vi "FPGA Combined.vi"() -> ()   [LabVIEW 2017]
uses:
  <vilib>/ni/Engine Simulation Toolkit (EST)/Version Token.ctl
  <vilib>/ni/Engine Simulation Toolkit (EST)/APU/Settings.ctl
  <vilib>/ni/Engine Simulation Toolkit (EST)/APU/Input.ctl
  <vilib>/ni/Engine Simulation Toolkit (EST)/APU/Output.ctl
  <vilib>/ni/Engine Simulation Toolkit (EST)/Analog Replay/Settings.ctl
  <vilib>/ni/Engine Simulation Toolkit (EST)/Analog Replay/Input.ctl
  <vilib>/ni/Engine Simulation Toolkit (EST)/Analog Replay/Load Input.ctl
  <vilib>/ni/Engine Simulation Toolkit (EST)/Digital Pattern Generation/Load Input.ctl
  <vilib>/ni/Engine Simulation Toolkit (EST)/Digital Pattern Generation/Settings.ctl
  <vilib>/ni/Engine Simulation Toolkit (EST)/Digital Pattern Generation/Input.ctl
  <vilib>/ni/Engine Simulation Toolkit (EST)/APU/Shared Settings.ctl
  Documents/github/NIVeristandAdd-ons/FPGA-Custom-Device/Source/FPGA/Speciality IO/Types/PWM.Generate.Digital.Settings.ctl
  Documents/github/NIVeristandAdd-ons/FPGA-Custom-Device/Source/FPGA/Speciality IO/Types/PWM.Measure.Digital.Settings.ctl
  Documents/github/NIVeristandAdd-ons/FPGA-Custom-Device/Source/FPGA/Speciality IO/Types/PWM.Measure.Digital.Measurement.ctl
  Documents/github/NIVeristandAdd-ons/FPGA-Custom-Device/Source/FPGA/Speciality IO/Types/Sine.Generate.Settings.ctl
  Documents/github/NIVeristandAdd-ons/FPGA-Custom-Device/Source/FPGA/Speciality IO/Types/PWM.Measure.Analog.Settings.ctl
  Documents/github/NIVeristandAdd-ons/FPGA-Custom-Device/Source/FPGA/Speciality IO/Types/PWM.Measure.Analog.Measurement.ctl
  <vilib>/Platform/TimedLoop/XDataNode/timing_clust.ctl
  <vilib>/Platform/TimedLoop/XDataNode/nitl_modes.ctl
  <vilib>/Platform/TimedLoop/XDataNode/wakeup.ctl
  <vilib>/rvi/Emulation/niFpgaGetClockAttributes.vi
  <vilib>/rvi/Emulation/niFpgaSctlEmulationGetInTimedLoop.vi
  <vilib>/rvi/Emulation/niFpgaEmulationReportErrorSimple.vi
  <vilib>/rvi/DataTransferAndStorage/Container/Common/niFpgaContainerGetUniqueNameForEmu.vi
  <vilib>/rvi/DataTransferAndStorage/Container/Common/niFpgaContainerSetEmuInfo.vi
  <vilib>/rvi/eio/common/nirviEmuReportErrorAndStop.vi
  <vilib>/rvi/Emulation/niFpgaCriticalErrorInLSC.vi
  <vilib>/rvi/eio/common/nirviEmuTemplateMethod_errors.vi
  <vilib>/rvi/Emulation/niFpgaProcessEmulError.vi
  <vilib>/Platform/TimedLoop/XDataNode/XDataNode.xnode
  <vilib>/rvi/LocalResourceManager/LocalResourceManager.xnode
  <vilib>/eio/EIONode/EIONode.xnode
  <vilib>/eio/EIOMethodNode/EIOMethodNode.xnode
  <vilib>/Platform/TimedLoop/XDataNode/XDNodeRunTimeDep.lvlib
  <vilib>/ni/Engine Simulation Toolkit (EST)/APU/APU.lvlib
  <vilib>/ni/Engine Simulation Toolkit (EST)/Analog Replay/Analog Replay.lvlib
  <vilib>/ni/Engine Simulation Toolkit (EST)/Digital Pattern Generation/Digital Pattern Generation.lvlib
  Documents/github/NIVeristandAdd-ons/FPGA-Custom-Device/Source/FPGA/Speciality IO/Speciality FPGA IO.lvlib
  <vilib>/NI Veristand/FPGA/NI_VS FPGA Support.lvlib
  <vilib>/ni/Engine Simulation Toolkit (EST)/Engine Simulation Toolkit.lvlib
panel:
  in  "_Low Pulse 0":u32
  in  "_High Pulse 0":u32
  in  "_Low Pulse 1":u32
  in  "_High Pulse 1":u32
  in  "_PWM In 0 timeout":u32=40000
  out "_PWM In 0 High Time":u32
  out "_PWM In 0 Low Time":u32
  in  "_PWM In 1 timeout":u32=40000
  out "_PWM In 1 High Time":u32
  out "_PWM In 1 Low Time":u32
  in  "Generate IRQ":bool
  in  "Clock Pulse":bool
  in  "Clock Ticked":bool
  in  "Use External Timing":bool
  in  "Write to  RTSI":bool
  in  "Loop Rate (usec)":u32
  in  "Start":bool
  out "Measure.Analog.Ch0":T1={"ACTIVE TICKS"=10, "INACTIVE TICKS"=10, "ACQ TICKS"=400, "ACTIVE VOLTAGE"=4.979251861572266, "INACTIVE VOLTAGE"=-4.979404449462891}
  out "Measure.Analog.Ch1":T1={"ACTIVE TICKS"=90, "INACTIVE TICKS"=10, "ACQ TICKS"=400, "ACTIVE VOLTAGE"=-6.998723030090332, "INACTIVE VOLTAGE"=6.998509407043457}
  in  "Measure.Analog.Ch0.Settings":T2={"ACTIVE EDGE"=TRUE, "TIMEOUT"=40000000, "THRESHOLD"=0.0}
  in  "Measure.Analog.Ch1.Settings":T2={"ACTIVE EDGE"=FALSE, "TIMEOUT"=40000000, "THRESHOLD"=95.0}
  out "Analog.Generation.Ticks 2":u32=10 caption="Count(uSec)"
  in  "Analog.Generation.Ticks":u32=10 caption="Count(uSec)"
  in  "Sine":bool=TRUE
  in  "Generate.Sine.Ch0.Settings":T3
  in  "Generate.Sine.Ch1.Settings":T3
  out "Measure.Digital.Ch0":T4={"ACTIVE TICKS"=4000, "INACTIVE TICKS"=12000, "ACQ TICKS"=1}
  out "Measure.Digital.Ch1":T4
  in  "Measure.Digital.Ch0.Settings":T5={"ACTIVE EDGE"=TRUE, "TIMEOUT"=40000000}
  in  "Measure.Digital.Ch1.Settings":T5={"ACTIVE EDGE"=FALSE, "TIMEOUT"=40000000}
  in  "Generate.Digital.Ch0.Internal.Settings":T6={"ACTIVE EDGE"=TRUE, "ACTIVE TICKS"=4000, "INACTIVE TICKS"=12000}
  in  "Generate.Digital.Ch1.Internal.Settings":T6={"ACTIVE EDGE"=FALSE, "ACTIVE TICKS"=60000000, "INACTIVE TICKS"=20000000}
  in  "shared settings.apu 1":T7 {"start" format="%#.15g"}
  in  "go.apu 1":bool
  in  "load input.Cam2 DIO 1":T8
  in  "input.Cam1 DIO 0":T9
  in  "settings.Cam1 DIO 0":T10
  in  "input.Cam2 DIO 1":T9
  in  "settings.Cam2 DIO 1":T10
  in  "load input.Cam1 DIO 0":T8
  in  "load input.Crank AO 0":T11={"Data"=[0, 0, 0, 0, 0, 0, 0, 0, 0, 0, 0, 0, 0, 0, 0, 0], "LoadOffset"=0, "Done"=FALSE} caption="input"
  in  "input.Crank AO 0":T12 caption="input"
  in  "settings.Crank AO 0":T13 caption="settings"
  out "output.apu 1":T14 caption="output"
  in  "input.apu 1":T15={"desired speed"=0.0, "reset"=TRUE} caption="input"
  in  "settings.apu 1":T16 caption="settings"
  in  "est.version":T17
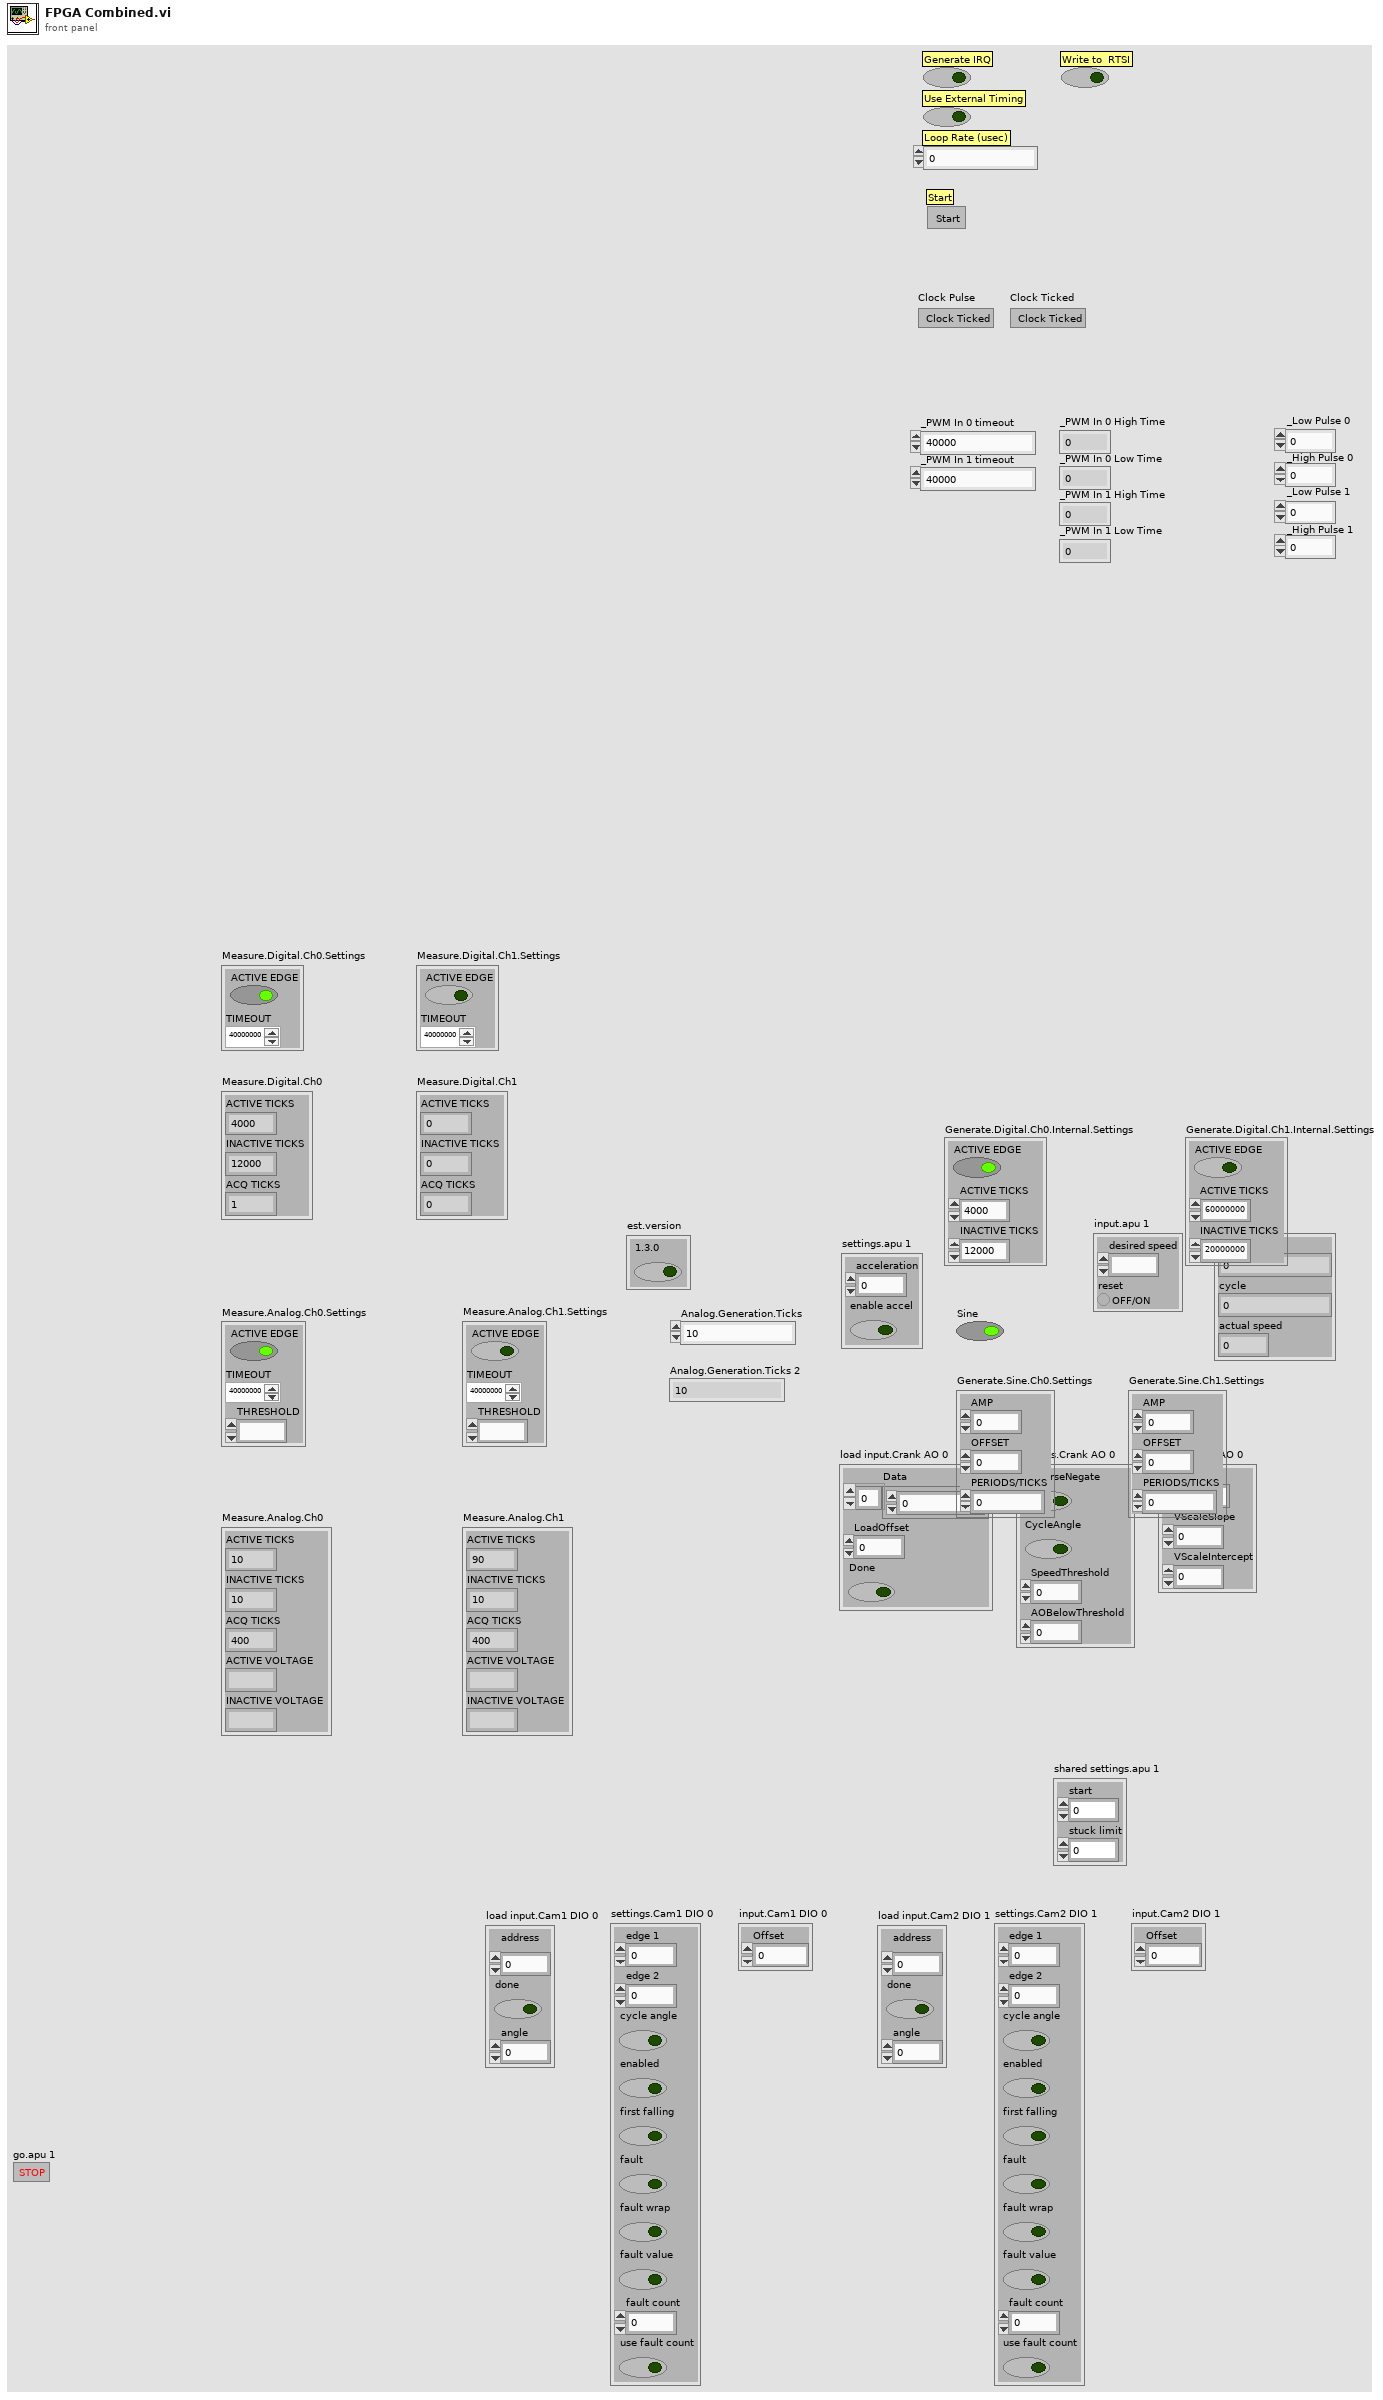
[diagram p1: front panel]
types:
  T1 = typedef "Speciality FPGA IO.lvlib/PWM.Measure.Analog.Measurement.ctl" = cluster{"ACTIVE TICKS":u32, "INACTIVE TICKS":u32, "ACQ TICKS":u32, "ACTIVE VOLTAGE":fxp<+/-,32,8>, "INACTIVE VOLTAGE":fxp<+/-,32,8>}
  T2 = typedef "Speciality FPGA IO.lvlib/PWM.Measure.Analog.Settings.ctl" = cluster{"ACTIVE EDGE":bool, "TIMEOUT":u32, "THRESHOLD":fxp<+/-,32,8>}
  T3 = typedef "Speciality FPGA IO.lvlib/Sine.Generate.Settings.ctl" = cluster{"AMP":fxp<+/-,32,8>, "OFFSET":fxp<+/-,32,8>, "PERIODS/TICKS":fxp<+,32,0>}
  T4 = typedef "Speciality FPGA IO.lvlib/PWM.Measure.Digital.Measurement.ctl" = cluster{"ACTIVE TICKS":u32, "INACTIVE TICKS":u32, "ACQ TICKS":u32}
  T5 = typedef "Speciality FPGA IO.lvlib/PWM.Measure.Digital.Settings.ctl" = cluster{"ACTIVE EDGE":bool, "TIMEOUT":u32}
  T6 = typedef "Speciality FPGA IO.lvlib/PWM.Generate.Digital.Settings.ctl" = cluster{"ACTIVE EDGE":bool, "ACTIVE TICKS":u32, "INACTIVE TICKS":u32}
  T7 = typedef "Engine Simulation Toolkit.lvlib/APU.lvlib/Shared Settings.ctl" = cluster{"start":fxp<+,17,17>, "stuck limit":fxp<+,18,18>}
  T8 = typedef "Engine Simulation Toolkit.lvlib/Digital Pattern Generation.lvlib/Load Input.ctl" = cluster{"address":fxp<+,11,11>, "done":bool, "angle":u16}
  T9 = typedef "Engine Simulation Toolkit.lvlib/Digital Pattern Generation.lvlib/Input.ctl" = cluster{"Offset":i16}
  T10 = typedef "Engine Simulation Toolkit.lvlib/Digital Pattern Generation.lvlib/Settings.ctl" = cluster{"edge 1":u16, "edge 2":u16, "cycle angle":bool, "enabled":bool, "first falling":bool, "fault":bool, "fault wrap":bool, "fault value":bool, "fault count":fxp<+,4,4>, "use fault count":bool}
  T11 = typedef "Engine Simulation Toolkit.lvlib/Analog Replay.lvlib/Load Input.ctl" = cluster{"Data":i16[], "LoadOffset":u16, "Done":bool}
  T12 = typedef "Engine Simulation Toolkit.lvlib/Analog Replay.lvlib/Input.ctl" = cluster{"Offset":i16, "VScaleSlope":fxp<+,18,6>, "VScaleIntercept":fxp<+/-,18,3>}
  T13 = typedef "Engine Simulation Toolkit.lvlib/Analog Replay.lvlib/Settings.ctl" = cluster{"ReverseNegate":bool, "CycleAngle":bool, "SpeedThreshold":fxp<+/-,23,2>, "AOBelowThreshold":i16}
  T14 = typedef "Engine Simulation Toolkit.lvlib/APU.lvlib/Output.ctl" = cluster{"crank":u16, "cycle":u16, "actual speed":fxp<+/-,23,2>}
  T15 = typedef "Engine Simulation Toolkit.lvlib/APU.lvlib/Input.ctl" = cluster{"desired speed":fxp<+/-,23,2>, "reset":bool}
  T16 = typedef "Engine Simulation Toolkit.lvlib/APU.lvlib/Settings.ctl" = cluster{"acceleration":fxp<+,18,-20>, "enable accel":bool}
  T17 = typedef "Engine Simulation Toolkit.lvlib/Version Token.ctl" = cluster{"1.3.0":bool}
  T18 = typedef "XDNodeRunTimeDep.lvlib/timing_clust.ctl" = cluster{"Expected End [f-1]":u64, "Actual End [f-1]":u64, "Finished Late? [f-1]":bool, "Expected End [i-1]":u64, "Actual End [i-1]":u64, "Finished Late? [i-1]":bool, "Expected Start [i]":u64, "Actual Start [i]":u64, "Expected Start [f]":u64, "Actual Start [f]":u64, "Source Name":string, "Structure Name":string, "Period":i64, "Deadline":i64, "Offset":i64, "Start":i64, "Priority":i32, "Timeout":i32, "Mode":T19, "Wakeup Reason":T20, "Error":errorcluster, "Source Type":string, "Secondary Source Type":string, "Global End Time":u64, "Global Start Time":u64, "Frame Duration":u64, "Iteration Duration":u64, "Assigned CPU":i32, "I/O Scan Engine Mode":u32}
  T19 = typedef "XDNodeRunTimeDep.lvlib/nitl_modes.ctl" = enum32{"No Change", "Process missed periods, maintain original phase", "Discard missed periods, maintain original phase", "Process missed periods, ignore original phase", "Discard missed periods, ignore original phase"}
  T20 = typedef "XDNodeRunTimeDep.lvlib/wakeup.ctl" = enum32{"Normal", "Aborted", "Asynchronous wakeup", "Timing source error", "Timed loop error", "Timeout"}
  T21 = typedef "Engine Simulation Toolkit.lvlib/APU.lvlib/Register Bus.ctl" = cluster{"Speed":refnum<k21>, "Crank Angle":refnum<k21>, "Cycle Angle":refnum<k21>, "Crank Count":refnum<k21>, "Cycle Count":refnum<k21>, "1.25 MHz Counter":refnum<k21>, "Crank Rollover":refnum<k21>, "Cycle Rollover":refnum<k21>, "shared settings":T7}
  T22 = typedef "Engine Simulation Toolkit.lvlib/Digital Pattern Generation.lvlib/Load Data.ctl" = cluster{"max address":fxp<+,11,11>, "memory":refnum<k21>}
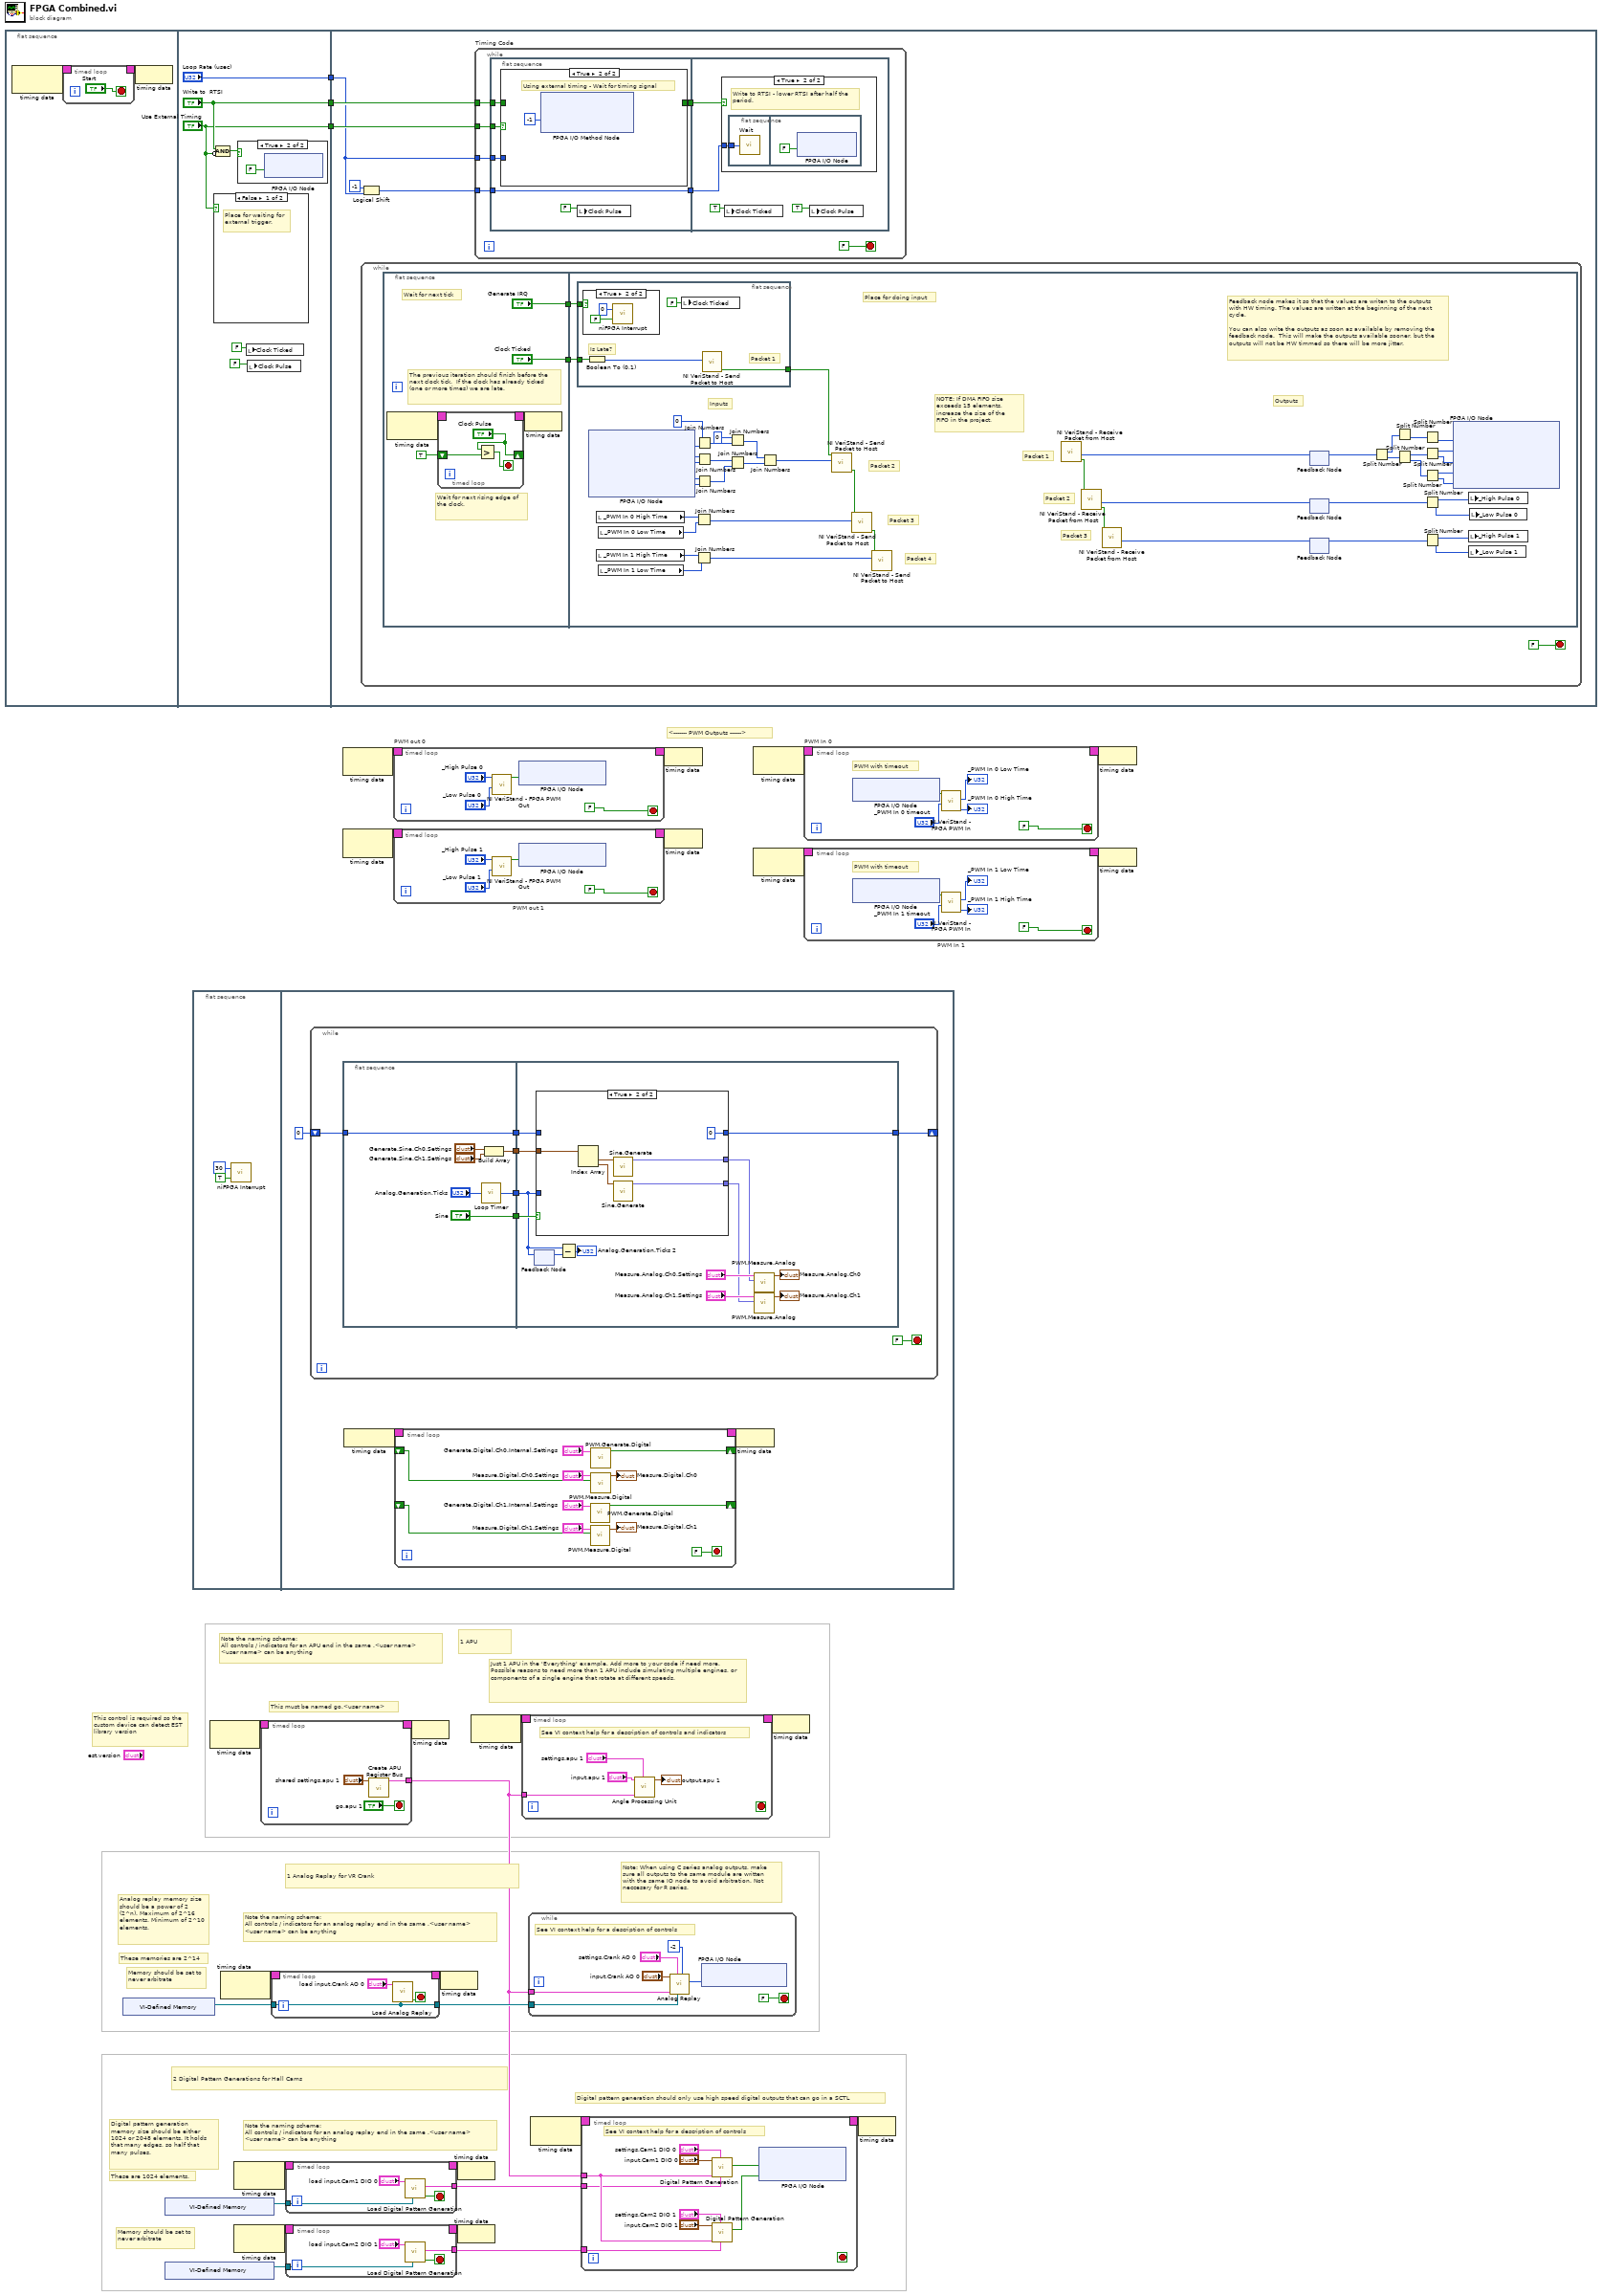
[diagram p0: block diagram]
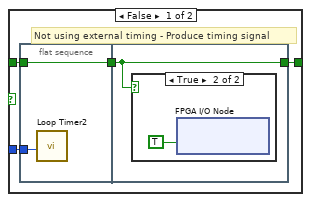
[diagram p4: hidden frame]
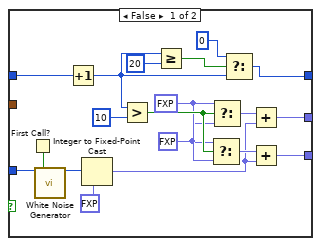
[diagram p8: hidden frame]
diagram:
  # "<------- PWM Outputs ------>"
  # "This must be named go.<user name>"
  # "Memory should be set to never arbitrate"
  # "Memory should be set to never arbitrate"
  # "Digital pattern generation should only use high speed digital outputs that can go in a SCTL"
  # "2 Digital Pattern Generations for Hall Cams"
  # "Note the naming scheme: \nAll controls / indicators for an analog replay end in the same .<user name>\n<user name> can be anything"
  # "These are 1024 elements."
  # "Digital pattern generation memory size should be either 1024 or 2048 elements. It holds that many edges, so half that many pulses."
  # "Note: When using C series analog outputs, make sure all outputs to the same module are written with the same IO node to avoid arbitration. Not neccesary for R series."
  # "1 Analog Replay for VR Crank"
  # "1 APU"
  # "These memories are 2^14"
  # "Note the naming scheme: \nAll controls / indicators for an APU end in the same .<user name>\n<user name> can be anything"
  # "Note the naming scheme: \nAll controls / indicators for an analog replay end in the same .<user name>\n<user name> can be anything"
  # "Analog replay memory size should be a power of 2 (2^n). Maximum of 2^16 elements. Minimum of 2^10 elements."
  # "Just 1 APU in the 'Everything' example. Add more to your code if need more. Possible reasons to need more than 1 APU include simulating multiple engines, or components of a single engine that rotate at different speeds."
  # "This control is required so the custom device can detect EST library version"
  n1 = flat-sequence {
    tunnel: ["Use External Timing"] -> w3
    tunnel: ["Write to  RTSI"] -> w2
    tunnel: ["Loop Rate (usec)"] -> w1
    tunnel: w3 -> [w47]
    tunnel: w2 -> [w46]
    tunnel: w1 -> [w45]
    frame #0 {
      n2 = node-c288() -> (w32:T18)  [unwired: 1 out]
      n3 = timed-loop {
        timing: w32 -> [_]
        timing-out: [_] -> w31
        stop <- "Start" stop-if-true
      }
      n4 = node-c288(w31) -> ()
    }
    frame #1 {
      n5 = case shown="False" "Use External Timing" {
        frame False {
          # "Place for waiting for external trigger."
        }
        frame True {
          # "Do not wait on trigger when externally timed."
        }
      }
      n6 = Compound Arithmetic op=AND("Write to  RTSI", invert "Use External Timing") -> (w42:bool)
      n7 = case shown="True" w42 {
        frame False {
        }
        frame True {
          n8 = xnode "FPGA I/O Node"("PXI_Trig0"=FALSE ("TRIG0")) -> ()  [unwired: 1 in, 1 out]
        }
      }
      n9 = local write "Clock Ticked"(FALSE ("Clock Ticked")) -> ()
      n10 = local write "Clock Pulse"(FALSE ("Clock Ticked")) -> ()
    }
    frame #2 {
      n11 = Logical Shift(y=i8 -1, x=w45) -> (x << y=w48:u32)
      n12 = while {
        stop <- FALSE stop-if-true
        n13 = flat-sequence {
          tunnel: ["Generate IRQ"] -> w80
          tunnel: ["Clock Ticked"] -> w79
          tunnel: w80 -> [w139]
          tunnel: w79 -> [w138]
          frame #0 {
            # "The previous iteration should finish before the next clock tick.  If the clock has already ticked (one or more times) we are late."
            # "Wait for next rising edge of the clock."
            # "Wait for next tick"
            n14 = node-c288() -> (w85:T18)  [unwired: 1 out]
            n15 = timed-loop {
              timing: w85 -> [_]
              timing-out: [_] -> w84
              shift-right: ["Clock Pulse"] -> _
              shift-left: TRUE ("Clock Ticked") -> [w89]
              stop <- w88 stop-if-true
              n16 = Greater?(x="Clock Pulse", y=w89) -> (0:w88:bool)
            }
            n17 = node-c288(w84) -> ()
          }
          frame #1 {
            # "Inputs"
            # "Outputs"
            # "Packet 4"
            # "Packet 3"
            # "Packet 2"
            # "Packet 3"
            # "Packet 2"
            # "Packet 1"
            # "NOTE: If DMA FIFO size exceeds 15 elements, increase the size of the FIFO in the project."
            # "Feedback node makes it so that the values are writen to the outputs with HW timing. The values are written at the beginning of the next cycle.  \n\nYou can also write the outputs as soon as available by removing the feedback node.  This will make the outputs available sooner, but the outputs will not be HW timmed so there will be more jitter."
            # "Place for doing input"
            n18 = flat-sequence {
              tunnel: w139 -> [w144]
              tunnel: [w142] -> w94
              tunnel: w138 -> [w140]
              frame #0 {
                # "Packet 1"
                # "Is Late?"
                n19 = case shown="True" w144 {
                  frame False {
                  }
                  frame True {
                    n20 = call <vilib>:"niFPGA Interrupt.vi"("Wait Until Cleared (F)"=FALSE ("Wait Until Cleared"), "IRQ Number (0)"=u8 0 ("IRQ Number")) -> ()  [unwired: 1 in]
                  }
                }
                n21 = Boolean To (0,1)(Boolean=w140) -> (0, 1=w143:i16)
                n22 = local write "Clock Ticked"(FALSE ("Clock Ticked")) -> ()
                n23 = call <vilib>:"NI VeriStand - Send Packet to Host.vi"("Element"=w143) -> ("Next"=w142:bool)  [unwired: 1 in, 9 out]
              }
            }
            n24 = xnode "FPGA I/O Node"() -> ("Connector1/DIOPORT3"=w137:u8, "Connector1/DIOPORT3"=w136:u8, "Connector1/DIOPORT2"=w135:u8, "Connector1/DIOPORT1"=w134:u8, "Connector1/DIOPORT0"=w133:u8)  [unwired: 5 in, 5 out]
            n25 = local read "_PWM In 0 High Time"() -> (w127:u32)
            n26 = local read "_PWM In 1 High Time"() -> (w125:u32)
            n27 = local read "_PWM In 0 Low Time"() -> (w126:u32)
            n28 = local read "_PWM In 1 Low Time"() -> (w124:u32)
            n29 = Join Numbers(hi=w127, lo=w126) -> ((hi.lo)=w106:u64)
            n30 = Join Numbers(hi=w125, lo=w124) -> ((hi.lo)=w105:u64)
            n31 = Join Numbers(hi=u8 0, lo=w137) -> ((hi.lo)=w132:u16)
            n32 = Join Numbers(hi=w136, lo=w135) -> ((hi.lo)=w131:u16)
            n33 = Join Numbers(hi=w134, lo=w133) -> ((hi.lo)=w130:u16)
            n34 = Join Numbers(hi=u16 0, lo=w132) -> ((hi.lo)=w129:u32)
            n35 = Join Numbers(hi=w131, lo=w130) -> ((hi.lo)=w128:u32)
            n36 = Join Numbers(hi=w129, lo=w128) -> ((hi.lo)=w107:u64)
            n37 = call <vilib>:"NI VeriStand - Send Packet to Host.vi"("Element"=w107, "Prev"=w94) -> ("Next"=w96:bool)  [unwired: 1 in, 8 out]
            n38 = call <vilib>:"NI VeriStand - Send Packet to Host.vi"("Element"=w106, "Prev"=w96) -> ("Next"=w95:bool)  [unwired: 1 in, 8 out]
            n39 = call <vilib>:"NI VeriStand - Send Packet to Host.vi"("Element"=w105, "Prev"=w95) -> ()  [unwired: 1 in, 9 out]
            n40 = call <vilib>:"NI VeriStand - Receive Packet from Host.vi"() -> ("Next"=w98:bool, "Element"=w104:u64)  [unwired: 2 in, 8 out]
            n41 = call <vilib>:"NI VeriStand - Receive Packet from Host.vi"("Prev"=w98) -> ("Next"=w97:bool, "Element"=w103:u64)  [unwired: 1 in, 8 out]
            n42 = call <vilib>:"NI VeriStand - Receive Packet from Host.vi"("Prev"=w97) -> ("Element"=w102:u64)  [unwired: 1 in, 9 out]
            n43 = feedback-in #1(w104) -> ()
            n44 = feedback #1() -> (w101:u64)  [unwired: 1 out]
            n45 = feedback-in #2(w103) -> ()
            n46 = feedback #2() -> (w100:u64)  [unwired: 1 out]
            n47 = feedback-in #3(w102) -> ()
            n48 = feedback #3() -> (w99:u64)  [unwired: 1 out]
            n49 = Split Number(x=w101) -> (hi(x)=w118:u32, lo(x)=w117:u32)
            n50 = Split Number(x=w118) -> (lo(x)=w119:u16)  [unwired: 1 out]
            n51 = Split Number(x=w117) -> (hi(x)=w121:u16, lo(x)=w120:u16)
            n52 = Split Number(x=w119) -> (lo(x)=w108:u8)  [unwired: 1 out]
            n53 = Split Number(x=w121) -> (hi(x)=w109:u8, lo(x)=w110:u8)
            n54 = Split Number(x=w120) -> (hi(x)=w111:u8, lo(x)=w112:u8)
            n55 = Split Number(x=w100) -> (hi(x)=w116:u32, lo(x)=w115:u32)
            n56 = Split Number(x=w99) -> (hi(x)=w114:u32, lo(x)=w113:u32)
            n57 = xnode "FPGA I/O Node"("Connector0/DIOPORT0"=w108, "Connector0/DIOPORT1"=w109, "Connector0/DIOPORT0"=w110, "Connector0/DIOPORT1"=w111, "Connector0/DIOPORT0"=w112) -> ()  [unwired: 5 in, 5 out]
            n58 = local write "_High Pulse 0"(w116) -> ()
            n59 = local write "_High Pulse 1"(w114) -> ()
            n60 = local write "_Low Pulse 1"(w113) -> ()
            n61 = local write "_Low Pulse 0"(w115) -> ()
          }
        }
      }
      n62 = while "Timing Code" {
        tunnel: w48 -> [w56]
        tunnel: w45 -> [w55]
        tunnel: w47 -> [w54]
        tunnel: w46 -> [w53]
        stop <- FALSE stop-if-true
        n63 = flat-sequence {
          tunnel: w56 -> [w59]
          tunnel: w55 -> [w62]
          tunnel: w54 -> [w61]
          tunnel: w53 -> [w60]
          tunnel: [w59] -> w51
          tunnel: [w57] -> w50
          tunnel: w51 -> [w75]
          tunnel: w50 -> [w72]
          frame #0 {
            n64 = case shown="True" w61 {
              tunnel: w62 -> [w66 _]
              tunnel: w60 -> [w64 _]
              tunnel: [w63 _] -> w57
              frame False {
                # "Not using external timing - Produce timing signal"
                n65 = flat-sequence {
                  tunnel: [w67] -> w65
                  tunnel: w66 -> [w68]
                  tunnel: w64 -> [w67]
                  tunnel: w65 -> [w69]
                  tunnel: [w69] -> w63
                  frame #0 {
                    n66 = call "Loop Timer2"("Count(uSec)"=w68) -> ()  [unwired: 1 out]
                  }
                  frame #1 {
                    n67 = case shown="True" w69 {
                      frame False {
                      }
                      frame True {
                        n68 = xnode "FPGA I/O Node"("PXI_Trig0"=TRUE ("TRIG0")) -> ()  [unwired: 1 in, 1 out]
                      }
                    }
                  }
                }
              }
              frame True {
                # "Using external timing - Wait for timing signal"
                n69 = xnode "FPGA I/O Method Node"("Timeout"=-1) -> ()  [unwired: 1 in, 2 out]
              }
            }
            n70 = local write "Clock Pulse"(FALSE ("Clock Ticked")) -> ()
          }
          frame #1 {
            n71 = case shown="True" w72 {
              tunnel: w75 -> [_ w76]
              frame False {
              }
              frame True {
                # "Write to RTSI - lower RTSI after half the period."
                n72 = flat-sequence {
                  tunnel: w76 -> [w77]
                  frame #0 {
                    n73 = call "Wait"("Count(uSec)"=w77) -> ()  [unwired: 1 out]
                  }
                  frame #1 {
                    n74 = xnode "FPGA I/O Node"("PXI_Trig0"=FALSE ("TRIG0")) -> ()  [unwired: 1 in, 1 out]
                  }
                }
              }
            }
            n75 = local write "Clock Ticked"(TRUE ("Clock Ticked")) -> ()
            n76 = local write "Clock Pulse"(TRUE ("Clock Ticked")) -> ()
          }
        }
      }
    }
  }
  n77 = xnode "VI-Defined Memory"() -> ("Memory Out"=w26:refnum<k21>)
  n78 = xnode "VI-Defined Memory"() -> ("Memory Out"=w20:refnum<k21>)
  n79 = xnode "VI-Defined Memory"() -> ("Memory Out"=w16:refnum<k21>)
  n80 = flat-sequence {
    frame #0 {
      n81 = call <vilib>:"niFPGA Interrupt.vi"("Wait Until Cleared (F)"=TRUE, "IRQ Number (0)"=u8 30) -> ()  [unwired: 1 in]
    }
    frame #1 {
      n82 = while {
        shift-right: [w171] -> _
        shift-left: i16 0 -> [w172]
        stop <- FALSE stop-if-true
        n83 = flat-sequence {
          tunnel: [w179] -> w173
          tunnel: w172 -> [w179]
          tunnel: [w178] -> w170
          tunnel: ["Sine"] -> w168
          tunnel: [w174] -> w167
          tunnel: w173 -> [w186]
          tunnel: [w187] -> w171
          tunnel: w170 -> [w182]
          tunnel: w168 -> [w185]
          tunnel: w167 -> [w184]
          frame #0 {
            n84 = call "Loop Timer"("Count(uSec)"="Analog.Generation.Ticks") -> ("Tick Count(uSec)"=w178:u32)
            n85 = Build Array("Generate.Sine.Ch0.Settings", "Generate.Sine.Ch1.Settings") -> (w174:T3[])
          }
          frame #1 {
            n86 = feedback-in #4(w182) -> ()
            n87 = feedback #4() -> (w183:u32)  [unwired: 1 in]
            n88 = case shown="True" w185 {
              tunnel: [w195 w213] -> w189
              tunnel: [w196 w214] -> w188
              tunnel: w186 -> [w199 _]
              tunnel: w182 -> [w198 _]
              tunnel: [w197 i16 0 ("t")] -> w187
              tunnel: w184 -> [_ w217]
              frame False {
                w206 = fxp<+/-,32,8> 12.0 ("t")
                w207 = fxp<+/-,32,8> -12.0 ("PWM")
                n89 = First Call?() -> (First Call?: T/F=w205:bool)
                n90 = call "White Noise Generator"("seed"=w198, "reset"=w205) -> ("white noise out"=w204:i16)  [unwired: 13 in]
                n91 = Increment(x=w199) -> (x+1=w209:i16)
                n92 = Integer to Fixed-Point Cast(fixed-point type=fxp<+/-,16,1> 0.0, integer=w204) -> (fixed-point=w194:fxp<+/-,16,1>)
                n93 = Greater?(x=w209, y=i16 10) -> (0:w208:bool)
                n94 = Greater Or Equal?(x=w209, y=i16 20) -> (x >= y?=w200:bool)
                n95 = Select(t=w206, s=w208, f=w207) -> (s? t:f=w201:fxp<+/-,32,8>)
                n96 = Select(t=w207, s=w208, f=w206) -> (s? t:f=w202:fxp<+/-,32,8>)
                n97 = Select(t=i16 0, s=w200, f=w209) -> (s? t:f=w197:i16)
                n98 = Add(x=w202, y=w194) -> (x+y=w196:fxp<+/-,33,9>)
                n99 = Add(x=w201, y=w194) -> (x+y=w195:fxp<+/-,33,9>)
              }
              frame True {
                n100 = Index Array(array=w217) -> (element #1=w216:T3, element #2=w215:T3)  [unwired: 2 in]
                n101 = call "Sine.Generate.vi"("Settings"=w216) -> ("Output"=w214:fxp<+/-,32,8>)  [unwired: 10 in]
                n102 = call "Sine.Generate.vi"("Settings"=w215) -> ("Output"=w213:fxp<+/-,32,8>)  [unwired: 10 in]
              }
            }
            n103 = Subtract(x=w182, y=w183) -> (x-y=→"Analog.Generation.Ticks 2":u32)
            n104 = call "PWM.Measure.Analog.vi"("PWM"=w188, "Settings"="Measure.Analog.Ch0.Settings") -> ("Measurement"=→"Measure.Analog.Ch0":T1)  [unwired: 8 in, 1 out]
            n105 = call "PWM.Measure.Analog.vi"("PWM"=w189, "Settings"="Measure.Analog.Ch1.Settings") -> ("Measurement"=→"Measure.Analog.Ch1":T1)  [unwired: 8 in, 1 out]
          }
        }
      }
      n106 = node-c288() -> (w151:T18)
      n107 = timed-loop {
        timing: w151 -> [_]
        timing-out: [_] -> w150
        shift-right: [w161] -> _
        shift-left: _ -> [w160]
        shift-right: [w159] -> _
        shift-left: _ -> [w158]
        stop <- FALSE stop-if-true
        n108 = call "PWM.Generate.Digital.vi"("Settings"="Generate.Digital.Ch1.Internal.Settings") -> ("Output"=w161:bool)  [unwired: 10 in]
        n109 = call "PWM.Measure.Digital.vi"("State"=w160, "Settings"="Measure.Digital.Ch1.Settings") -> ("Measurement"=→"Measure.Digital.Ch1":T4)  [unwired: 8 in, 1 out]
        n110 = call "PWM.Generate.Digital.vi"("Settings"="Generate.Digital.Ch0.Internal.Settings") -> ("Output"=w159:bool)  [unwired: 10 in]
        n111 = call "PWM.Measure.Digital.vi"("State"=w158, "Settings"="Measure.Digital.Ch0.Settings") -> ("Measurement"=→"Measure.Digital.Ch0":T4)  [unwired: 8 in, 1 out]
      }
      n112 = node-c288(w150) -> ()
    }
  }
  n113 = node-c288() -> (w14:T18)  [unwired: 1 in]
  n114 = node-c288() -> (w28:T18)  [unwired: 1 in]
  n115 = node-c288() -> (w24:T18)  [unwired: 1 in]
  n116 = node-c288() -> (w18:T18)  [unwired: 1 in]
  n117 = timed-loop {
    timing: w14 -> [_]
    timing-out: [_] -> w13
    tunnel: [w220] -> w12
    stop <- "go.apu 1" stop-if-true
    n118 = call <vilib>:"Create APU Register Bus.vi"("shared settings.<user name>"="shared settings.apu 1") -> ("register bus"=w220:T21)  [unwired: 10 in]
  }
  n119 = timed-loop {
    timing: w28 -> [_]
    timing-out: [_] -> w27
    tunnel: w26 -> [w224]
    tunnel: [w224] -> w25
    stop <- w225 stop-if-true
    n120 = call <vilib>:"Load Analog Replay.vi"("memory"=w224, "load input.<user name>"="load input.Crank AO 0") -> ("done"=w225:bool)  [unwired: 9 in]
  }
  n121 = timed-loop {
    timing: w24 -> [_]
    timing-out: [_] -> w23
    tunnel: w20 -> [w231]
    tunnel: [w230] -> w19
    stop <- w232 stop-if-true
    n122 = call <vilib>:"Load Digital Pattern Generation.vi"("memory"=w231, "load input.<user name>"="load input.Cam1 DIO 0") -> ("done"=w232:bool, "load data"=w230:T22)  [unwired: 8 in]
  }
  n123 = timed-loop {
    timing: w18 -> [_]
    timing-out: [_] -> w17
    tunnel: w16 -> [w237]
    tunnel: [w236] -> w15
    stop <- w238 stop-if-true
    n124 = call <vilib>:"Load Digital Pattern Generation.vi"("memory"=w237, "load input.<user name>"="load input.Cam2 DIO 1") -> ("done"=w238:bool, "load data"=w236:T22)  [unwired: 8 in]
  }
  n125 = node-c288() -> (w11:T18)  [unwired: 1 out]
  n126 = node-c288() -> (w9:T18)  [unwired: 1 out]
  n127 = timed-loop "PWM out 0" {
    timing: w11 -> [_]
    timing-out: [_] -> w10
    stop <- FALSE stop-if-true
    n128 = call <vilib>:"NI VeriStand - FPGA PWM Out.vi"("_Low Time"="_Low Pulse 0", "_High Time"="_High Pulse 0") -> ("Output"=w243:bool)  [unwired: 1 in, 8 out]
    n129 = xnode "FPGA I/O Node"("Connector0/DIO4"=w243) -> ()  [unwired: 1 in, 1 out]
  }
  n130 = timed-loop "PWM out 1" {
    timing: w9 -> [_]
    timing-out: [_] -> w8
    stop <- FALSE stop-if-true
    n131 = call <vilib>:"NI VeriStand - FPGA PWM Out.vi"("_Low Time"="_Low Pulse 1", "_High Time"="_High Pulse 1") -> ("Output"=w247:bool)  [unwired: 1 in, 8 out]
    n132 = xnode "FPGA I/O Node"("Connector0/DIO5"=w247) -> ()  [unwired: 1 in, 1 out]
  }
  n133 = node-c288(w13) -> ()
  n134 = node-c288(w27) -> ()
  n135 = node-c288(w23) -> ()
  n136 = node-c288(w17) -> ()
  n137 = node-c288() -> (w30:T18)  [unwired: 1 in]
  n138 = timed-loop {
    timing: w30 -> [_]
    timing-out: [_] -> w29
    tunnel: w12 -> [w253]
    stop <- _ stop-if-true
    # "See VI context help for a description of controls and indicators"
    n139 = call <vilib>:"Angle Processing Unit.vi"("settings.<user name>"="settings.apu 1", "register bus"=w253, "input.<user name>"="input.apu 1") -> ("output.<user name>"=→"output.apu 1":T14)  [unwired: 8 in]
  }
  n140 = while {
    tunnel: w25 -> [w265]
    tunnel: w12 -> [w259]
    stop <- FALSE stop-if-true
    # "See VI context help for a description of controls"
    n141 = call <vilib>:"Analog Replay.vi"("shift"=i8 -2, "memory"=w265, "settings.<user name>"="settings.Crank AO 0", "register bus"=w259, "input.<user name>"="input.Crank AO 0") -> ("analog value"=w260:i16)  [unwired: 6 in]
    n142 = xnode "FPGA I/O Node"("Connector0/AO0"=w260) -> ()  [unwired: 1 in, 1 out]
  }
  n143 = node-c288() -> (w22:T18)  [unwired: 1 in]
  n144 = timed-loop {
    tunnel: w12 -> [w268]
    timing: w22 -> [_]
    timing-out: [_] -> w21
    tunnel: w19 -> [w267]
    tunnel: w15 -> [w266]
    stop <- _ stop-if-true
    # "See VI context help for a description of controls"
    n145 = call <vilib>:"Digital Pattern Generation.vi"("load data"=w267, "settings.<user name>"="settings.Cam1 DIO 0", "register bus"=w268, "input.<user name>"="input.Cam1 DIO 0") -> ("digial output"=w271:bool)  [unwired: 7 in]
    n146 = call <vilib>:"Digital Pattern Generation.vi"("load data"=w266, "settings.<user name>"="settings.Cam2 DIO 1", "register bus"=w268, "input.<user name>"="input.Cam2 DIO 1") -> ("digial output"=w272:bool)  [unwired: 7 in]
    n147 = xnode "FPGA I/O Node"("Connector0/DIO0"=w271, "Connector0/DIO1"=w272) -> ()  [unwired: 2 in, 2 out]
  }
  n148 = node-c288(w10) -> ()
  n149 = node-c288(w8) -> ()
  n150 = node-c288() -> (w7:T18)  [unwired: 1 out]
  n151 = node-c288() -> (w5:T18)  [unwired: 1 out]
  n152 = node-c288(w29) -> ()
  n153 = timed-loop "PWM In 0" {
    timing: w7 -> [_]
    timing-out: [_] -> w6
    stop <- FALSE stop-if-true
    # "PWM with timeout"
    n154 = xnode "FPGA I/O Node"() -> ("Connector0/DIO0"=w280:bool)  [unwired: 1 in, 1 out]
    n155 = call <vilib>:"NI VeriStand - FPGA PWM In.vi"("Time Out"="_PWM In 0 timeout", "Value"=w280) -> ("High time"=→"_PWM In 0 High Time":u32, "Low Time"=→"_PWM In 0 Low Time":u32)  [unwired: 8 out]
  }
  n156 = timed-loop "PWM In 1" {
    timing: w5 -> [_]
    timing-out: [_] -> w4
    stop <- FALSE stop-if-true
    # "PWM with timeout"
    n157 = xnode "FPGA I/O Node"() -> ("Connector0/DIO1"=w287:bool)  [unwired: 1 in, 1 out]
    n158 = call <vilib>:"NI VeriStand - FPGA PWM In.vi"("Time Out"="_PWM In 1 timeout", "Value"=w287) -> ("High time"=→"_PWM In 1 High Time":u32, "Low Time"=→"_PWM In 1 Low Time":u32)  [unwired: 8 out]
  }
  n159 = node-c288(w21) -> ()
  n160 = node-c288(w6) -> ()
  n161 = node-c288(w4) -> ()
